vi "TCP Data read (SubVI).vi"(8 "error in (no error)":errorcluster, 10 "Запись в файл":bool, 11 "TCP Network Connection in":refnum<k5>) -> (0 "error out":errorcluster, 1 "Запись в файл вых":bool, 2 "Read data":string, 3 "TCP Network Connection out":refnum<k5>)   [LabVIEW 2013]
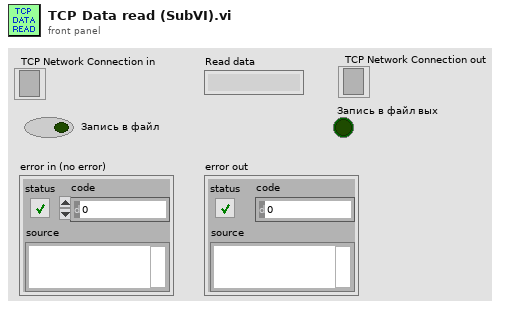
[diagram p1: front panel]
types:
  T1 = enum16{"Standard", "Buffered", "CRLF", "Immediate"}
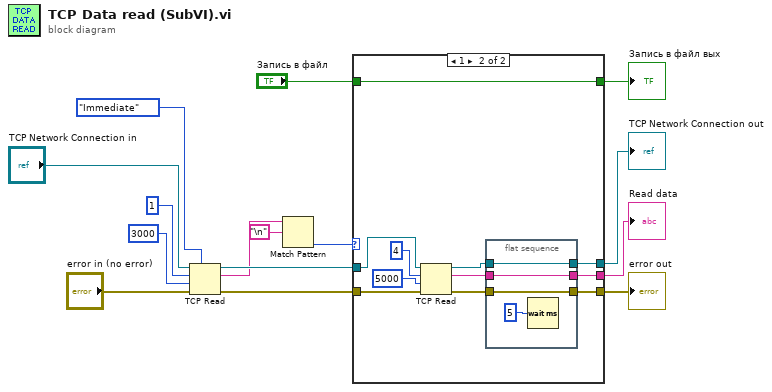
[diagram p0: block diagram]
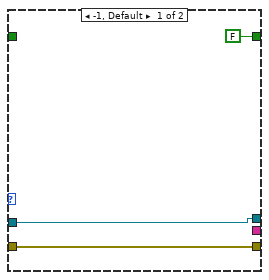
[diagram p2: hidden frame]
diagram:
  n1 = TCP Read(connection ID="TCP Network Connection in", bytes to read=1, error in (no error)="error in (no error)", 7:T1."Immediate" ("mode (standard)"), 9:3000 ("timeout ms (25000)")) -> (connection ID out=w4:refnum<k5>, data out=w3:string, error out=w12:errorcluster)
  n2 = Match Pattern(string=w3, regular expression="\n") -> (offset past match=w7:i32)  [unwired: 4 out]
  n3 = case shown="1" w7 {
    tunnel: [w18 w29] -> w14
    tunnel: [_ w28] -> w15
    tunnel: w4 -> [w16 w27]
    tunnel: "Запись в файл" -> [_ w21]
    tunnel: w12 -> [w18 w26]
    tunnel: [FALSE ("Запись в файл") w21] -> w2
    tunnel: [w16 w19] -> w1
    frame -1, Default {
    }
    frame 1 {
      n4 = TCP Read(connection ID=w27, bytes to read=4, error in (no error)=w26, 9:5000 ("timeout ms (25000)")) -> (connection ID out=w20:refnum<k5>, data out=w22:string, error out=w23:errorcluster)  [unwired: 1 out]
      n5 = flat-sequence {
        tunnel: w23 -> [w32]
        tunnel: [w32] -> w29
        tunnel: [w31] -> w28
        tunnel: w22 -> [w31]
        tunnel: w20 -> [w30]
        tunnel: [w30] -> w19
        frame #0 {
          n6 = Wait (ms)(milliseconds to wait=u32 5) -> ()  [unwired: 1 out]
        }
      }
    }
  }
  "Read data" <- w15
  "error out" <- w14
  "Запись в файл вых" <- w2
  "TCP Network Connection out" <- w1
